vi "1-InitialAllFunctionVIs.vi"(8 "error in (no error)":errorcluster, 11 "AllControls IN":T1) -> (0 "error out":errorcluster, 3 "AllControls Out":T1)   [LabVIEW 2017]
uses:
  Ctrls/AllControls.ctl
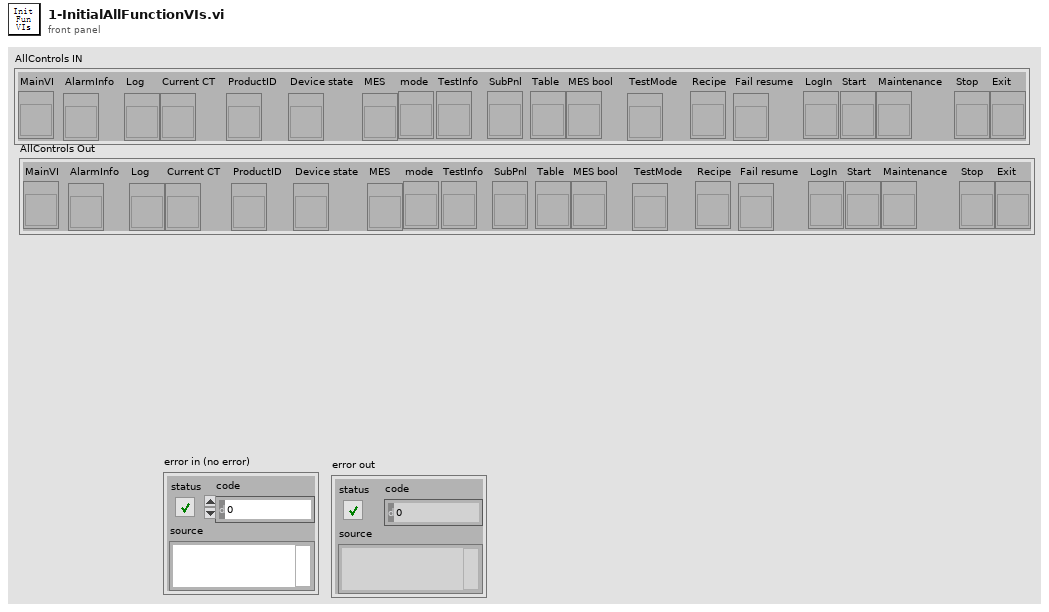
[diagram p1: front panel]
types:
  T1 = typedef "AllControls.ctl" = cluster{"MainVI":refnum<vi>, "AlarmInfo":refnum<vi>, "Log":refnum<vi>, "Current CT":refnum<vi>, "ProductID":refnum<vi>, "Device state":refnum<vi>, "MES":refnum<vi>, "mode":refnum<vi>, "TestInfo":refnum<vi>, "SubPnl":refnum<vi>, "Table":refnum<vi>, "MES bool":refnum<vi>, "TestMode":refnum<vi>, "Recipe":refnum<vi>, "Fail resume":refnum<vi>, "LogIn":refnum<vi>, "Start":refnum<vi>, "Maintenance":refnum<vi>, "Stop":refnum<vi>, "Exit":refnum<vi>}
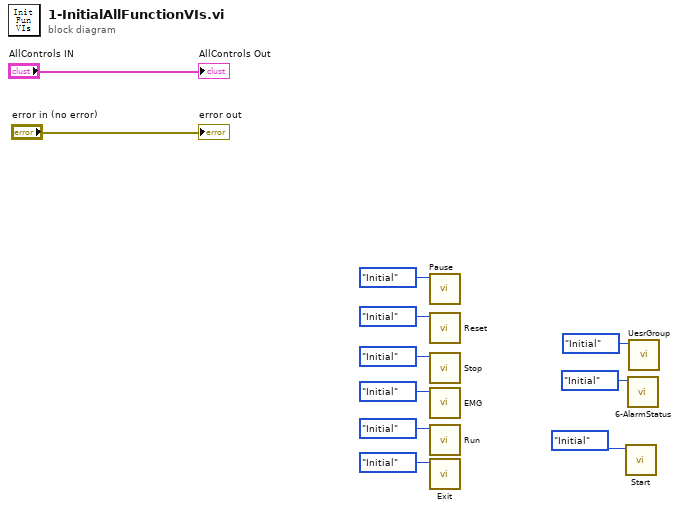
[diagram p0: block diagram]
diagram:
  n1 = call "Pause.vi"("Step"=enum16{"Initial", "Write", "Read"}."Initial") -> ()  [unwired: 9 in, 2 out]
  n2 = call "Reset.vi"("Step"=enum16{"Initial", "Write", "Read"}."Initial") -> ()  [unwired: 9 in, 2 out]
  n3 = call "Stop.vi"("Step"=enum16{"Initial", "Write", "Read"}."Initial") -> ()  [unwired: 9 in, 2 out]
  n4 = call "EMG.vi"("Step"=enum16{"Initial", "Write", "Read"}."Initial") -> ()  [unwired: 9 in, 2 out]
  n5 = call "Run.vi"("Step"=enum16{"Initial", "Write", "Read"}."Initial") -> ()  [unwired: 9 in, 2 out]
  n6 = call "Exit.vi"("Step"=enum16{"Initial", "Write", "Read"}."Initial") -> ()  [unwired: 9 in, 2 out]
  n7 = call "Start.vi"("Step"=enum16{"Initial", "Write", "Read"}."Initial") -> ()  [unwired: 9 in, 2 out]
  n8 = call "6-AlarmStatus.vi"("Step"=enum16{"Initial", "Write", "Read"}."Initial") -> ()  [unwired: 9 in, 2 out]
  n9 = call "UesrGroup.vi"("Step"=enum16{"Initial", "Write", "Read"}."Initial") -> ()  [unwired: 9 in, 2 out]
  "AllControls Out" <- "AllControls IN"
  "error out" <- "error in (no error)"
